vi "NR Fetch ModAcc.vi"(0 "RFmx Handle In":refnum<k21>, 1 "Selector String":string, 11 "error in (no error)":errorcluster) -> (4 "RFmx Handle Out":refnum<k21>, 6 "ModAcc Results":T1, 15 "error out":errorcluster)   [LabVIEW 2016, in "RFmxNR.lvlib"]
uses:
  RFmxNR.lvlib
  Typedefs/NR ModAcc Results.ctl
  Typedefs/NR ModAcc Component Carrier Results.ctl
  <resource>/objmgr/RFmxNR.rc
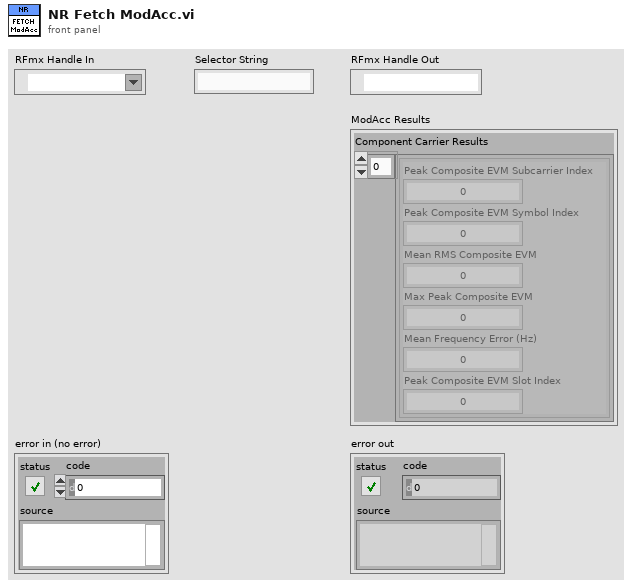
[diagram p1: front panel]
types:
  T1 = typedef "RFmxNR.lvlib/NR ModAcc Results.ctl" = cluster{"Component Carrier Results":T2[]}
  T2 = typedef "RFmxNR.lvlib/NR ModAcc Component Carrier Results.ctl" = cluster{"Peak Composite EVM Subcarrier Index":i32, "Peak Composite EVM Symbol Index":i32, "Mean RMS Composite EVM":dbl, "Max Peak Composite EVM":dbl, "Mean Frequency Error (Hz)":dbl, "Peak Composite EVM Slot Index":i32}
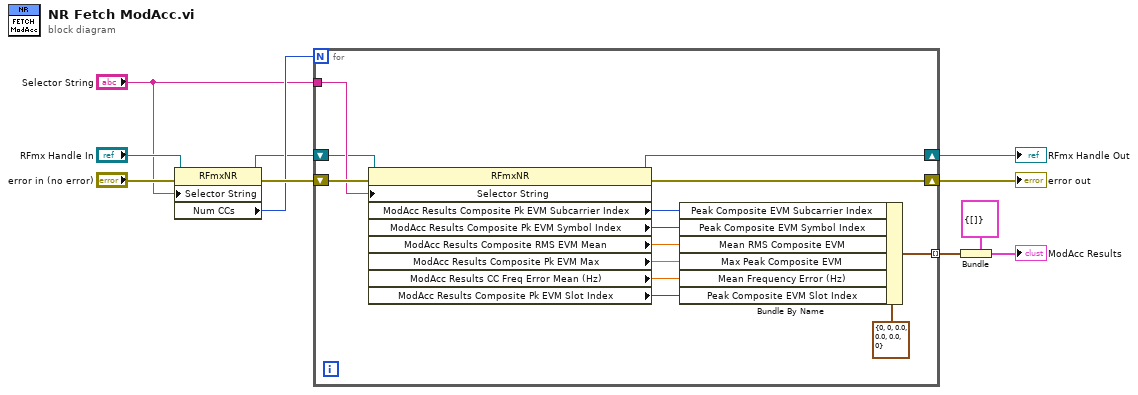
[diagram p0: block diagram]
diagram:
  n1 = property class="RFmxNR"(reference="RFmx Handle In", error in="error in (no error)", "Selector String"="Selector String") -> (reference out=w6:refnum<k21>, error out=w9:errorcluster, "Num CCs"=w8:i32)
  n2 = for {
    N: w8 -> [_]
    tunnel: "Selector String" -> [w23]
    shift-right: [w22] -> w7
    shift-left: w6 -> [w21]
    shift-right: [w20] -> w5
    shift-left: w9 -> [w24]
    tunnel: [w12] -> w3 mode=indexing
    n3 = property class="RFmxNR"(reference=w21, error in=w24, "Selector String"=w23) -> (reference out=w22:refnum<k21>, error out=w20:errorcluster, "ModAcc Results Composite Pk EVM Subcarrier Index"=w18:i32, "ModAcc Results Composite Pk EVM Symbol Index"=w17:i32, "ModAcc Results Composite RMS EVM Mean"=w16:dbl, "ModAcc Results Composite Pk EVM Max"=w15:dbl, "ModAcc Results CC Freq Error Mean (Hz)"=w14:dbl, "ModAcc Results Composite Pk EVM Slot Index"=w13:i32)
    n4 = Bundle By Name(cluster=T2 {"Peak Composite EVM Subcarrier Index"=0, "Peak Composite EVM Symbol Index"=0, "Mean RMS Composite EVM"=0.0, "Max Peak Composite EVM"=0.0, "Mean Frequency Error (Hz)"=0.0, "Peak Composite EVM Slot Index"=0} ("NR ModAcc Component Carrier Results"), "Peak Composite EVM Subcarrier Index"=w18, "Peak Composite EVM Symbol Index"=w17, "Mean RMS Composite EVM"=w16, "Max Peak Composite EVM"=w15, "Mean Frequency Error (Hz)"=w14, "Peak Composite EVM Slot Index"=w13) -> (w12:T2)
  }
  "error out" <- w5
  "RFmx Handle Out" <- w7
  n5 = Bundle(cluster=T1 {"Component Carrier Results"=[]} ("NR ModAcc Results"), "Component Carrier Results"=w3) -> (→"ModAcc Results":T1)
